vi "Nyquist Plot.vi"() -> ()   [LabVIEW 2018]
uses:
  <vilib>/addons/Control Design/_Model Construction/Model Typedefs.llb/CD Transfer Function Model (SISO).ctl
  <vilib>/addons/Control Design/_Model Construction/Data Typedefs.llb/CD frequency specs.ctl
  <vilib>/addons/Control Design/_Model Construction/Model Typedefs.llb/CD Transfer Function Model (MIMO).ctl
  <vilib>/addons/Control Design/_Model Construction/Model Typedefs.llb/CD General Elements.ctl
  <vilib>/addons/Control Design/_Utility/Rendering.llb/Rendering Transfer Function Options.ctl
  <vilib>/addons/Control Design/_Frequency Response Analysis/Frequency Response.llb/Frequency Response subVI/cd_Nyquist (Transfer Function).vi
  <vilib>/addons/Control Design/_Frequency Response Analysis/Frequency Response.llb/Frequency Response subVI/cd_Gain and Phase Margin (Transfer Function).vi
  <vilib>/addons/Control Design/_Utility/Model Viewer.llb/Model Viewer SubVI/cd_Draw Transfer Function Equation (TF).vi
  <vilib>/addons/Control Design/_Frequency Response Analysis/NI_CD_Frequency Response.lvlib
  <vilib>/addons/Control Design/_Model Construction/NI_LinSys_Data Typedefs.lvlib
  <vilib>/addons/Control Design/_Model Construction/NI_LinSys_Model Typedefs.lvlib
  <vilib>/addons/Control Design/_Utility/NI_CD_Model Viewer.lvlib
  <vilib>/addons/Control Design/_Utility/NI_LinSys_Rendering.lvlib
panel:
  out "nDelay":dbl
  out "P.M. Freq (rad/s)":dbl format="%#.2f"
  out "Phase Margin (rad)":dbl format="%#.2f"
  out "G.M. Freq (rad/s)":dbl format="%#.2f"
  out "Gain Margin":dbl format="%#.2f"
  out "Delay Margin":dbl format="%#.3f"
  out "D.M. Freq (rad/s)":dbl format="%#.2f"
  out "Forward Loop Transfer Function":picture
  in  "Transfer Function":T1[][](array[typedef]) {"delay" format="%.4f"; "Denominator" format="%#_6f"; "Numerator" format="%#.5f"}
  out "Nyquist Plot":cluster{"W":dbl[], "Magnitude":dbl[]}[](graph)
  # "Controls Board"
  # "Nyquist Plot"
  # "b0"
  # "b1"
  # "b2"
  # "b3"
  # "a0"
  # "a1"
  # "a2"
  # "a3"
  # "h"
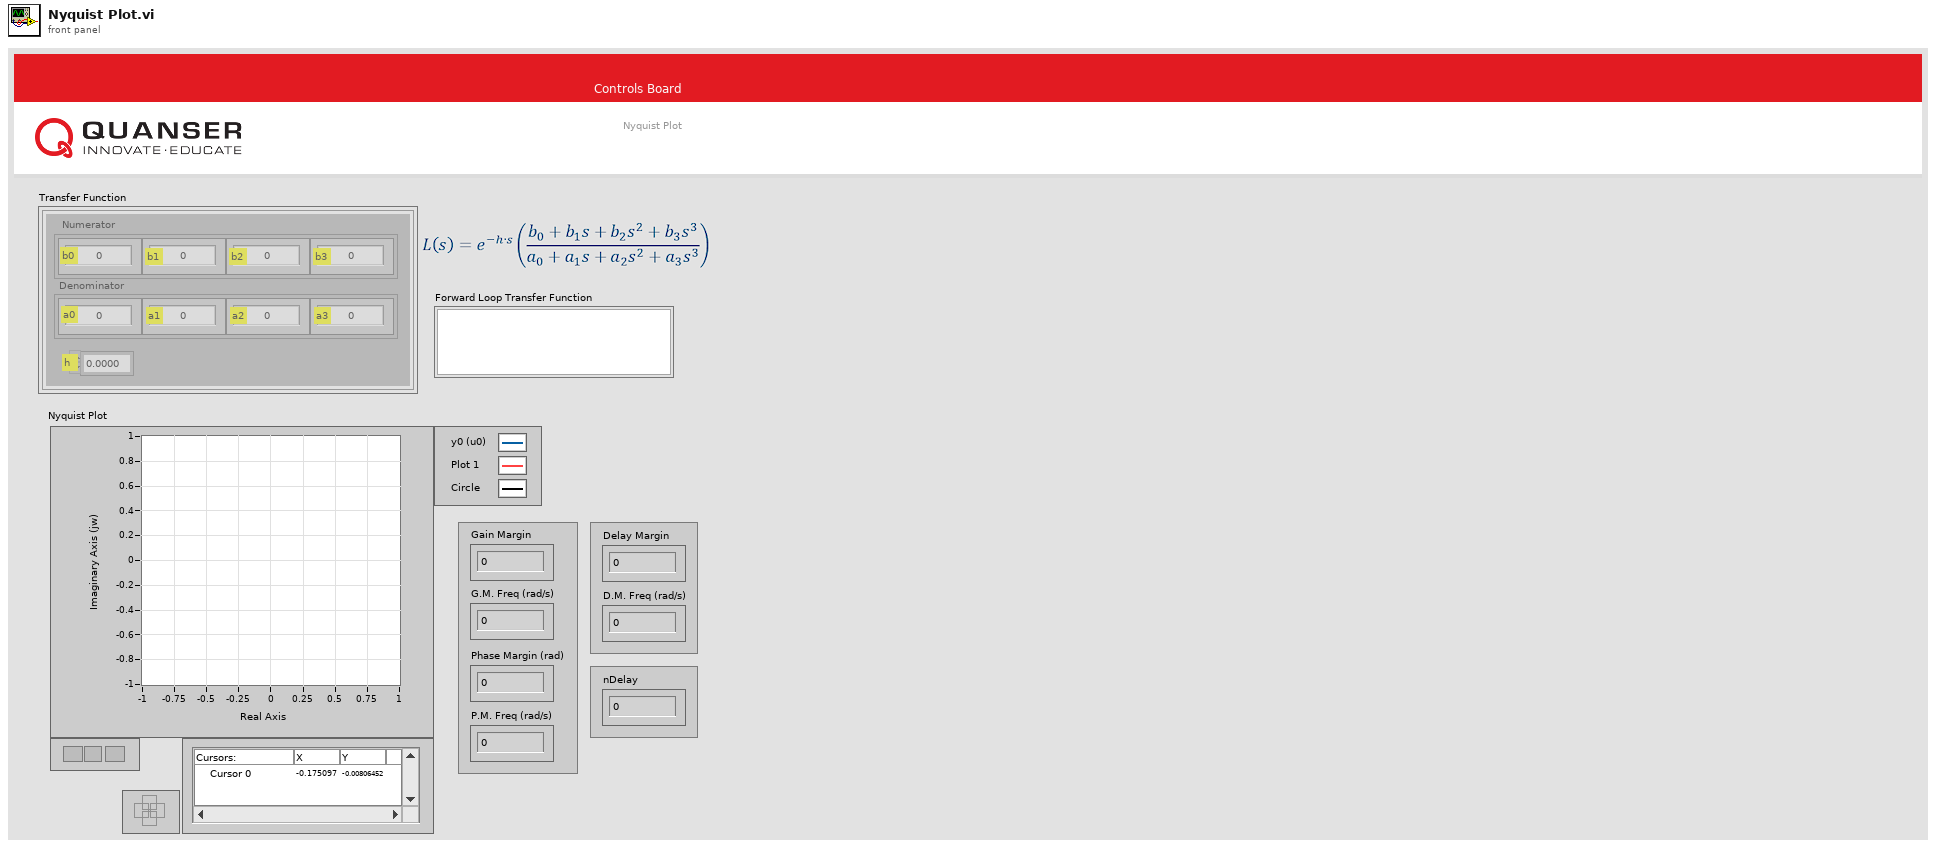
[diagram p1: front panel]
types:
  T1 = typedef "NI_LinSys_Model Typedefs.lvlib/CD Transfer Function Model (SISO).ctl" = cluster{"Numerator":dbl[], "Denominator":dbl[], "delay":dbl}
  T2 = typedef "NI_LinSys_Rendering.lvlib/Rendering Transfer Function Options.ctl" = u16
  T3 = typedef "NI_LinSys_Model Typedefs.lvlib/CD General Elements.ctl" = cluster{"Model name":string, "Input names":string[], "Output names":string[], "Input Delays":dbl[], "Output Delays":dbl[], "Sampling Time":dbl, "Notes":string}
  T4 = typedef "NI_LinSys_Model Typedefs.lvlib/CD Transfer Function Model (MIMO).ctl" = cluster{"properties":T3, "transfer function(s)":T1[][]}
  T5 = typedef "NI_LinSys_Data Typedefs.lvlib/CD frequency specs.ctl" = cluster{"Initial frequency":dbl, "Final frequency":dbl, "Minimum number of points":i32, "Frequency Unit":enum16{"Hz", "rad/s"}}
  T6 = typedef "NI_LinSys_Data Typedefs.lvlib/CD Margin Data.ctl" = cluster{"G.M. Frequency":dbl, "Gain Margin":dbl, "P.M. Frequency":dbl, "Phase Margin":dbl}
  T7 = typedef "NI_LinSys_Data Typedefs.lvlib/CD Delay Margin.ctl" = cluster{"D.M. Frequency":dbl, "Delay Margin":dbl}
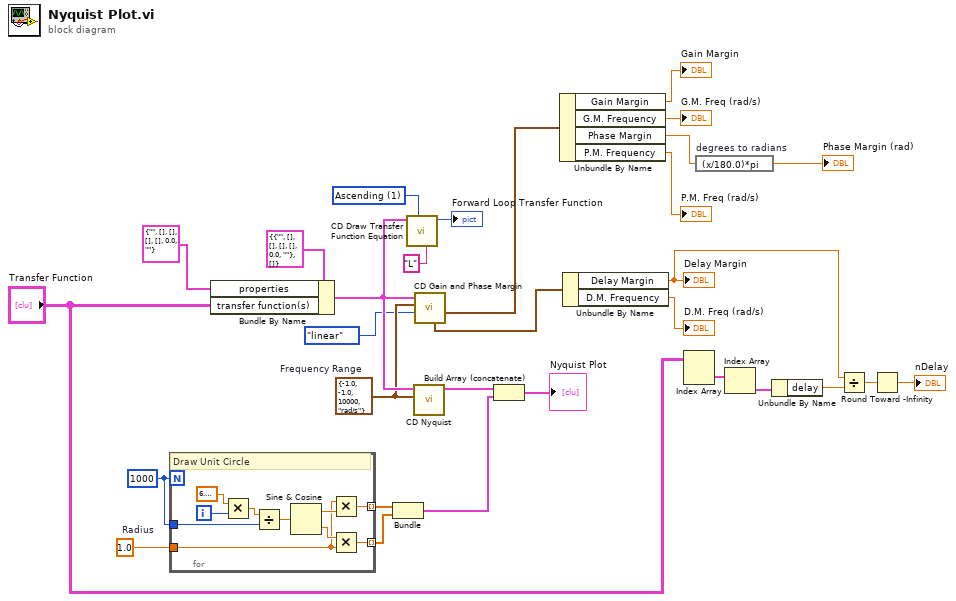
[diagram p0: block diagram]
diagram:
  w20 = T2 1 items=["Descending", "Ascending", "Negative Power"] ("Display Format")
  w24 = 1.0  # Radius
  w27 = 1000
  w18 = T5 {"Initial frequency"=-1.0, "Final frequency"=-1.0, "Minimum number of points"=10000, "Frequency Unit"=enum."rad/s"}  # Frequency Range
  n1 = for {
    N: w27 -> [_]
    tunnel: w27 -> [w38]
    tunnel: [w32] -> w26 mode=indexing
    tunnel: [w31] -> w25 mode=indexing
    tunnel: w24 -> [w33]
    i -> [w36]
    # "Draw Unit Circle"
    n2 = Multiply(x=6.283185307179586, y=w36) -> (x*y=w40:dbl)
    n3 = Divide(x=w40, y=w38) -> (x/y=w39:dbl)
    n4 = Sine & Cosine(0:w39) -> (1:w35:dbl, 2:w34:dbl)
    n5 = Multiply(x=w33, y=w35) -> (x*y=w32:dbl)
    n6 = Multiply(x=w34, y=w33) -> (x*y=w31:dbl)
  }
  n7 = Bundle By Name(cluster=T4 {"properties"={"Model name"="", "Input names"=[], "Output names"=[], "Input Delays"=[], "Output Delays"=[], "Sampling Time"=0.0, "Notes"=""}, "transfer function(s)"=[]} ("Transfer Function Model"), "properties"=T3 {"Model name"="", "Input names"=[], "Output names"=[], "Input Delays"=[], "Output Delays"=[], "Sampling Time"=0.0, "Notes"=""}, "transfer function(s)"="Transfer Function") -> (w19:T4)
  n8 = Bundle(w26, w25) -> (w22:cluster{dbl[], dbl[]})  [unwired: 1 in]
  n9 = call-poly <vilib>:"CD Draw Transfer Function Equation.vi"("Function Name (empty)"="L", "Display Format"=w20, "Transfer Function Model"=w19) -> ("Equation"=→"Forward Loop Transfer Function":picture)  [unwired: 6 in, 2 out]
  n10 = call-poly <vilib>:"CD Nyquist.vi"("Frequency Range"=w18, "Transfer Function Model"=w19) -> ("Nyquist Plot"=w23:cluster{"W":dbl[], "Magnitude":dbl[]}[])  [unwired: 7 in, 2 out]
  n11 = call-poly <vilib>:"CD Gain and Phase Margin.vi"("Magnitude Scale"=enum16{"linear", "dB"}."linear", "Frequency Range"=w18, "Transfer Function Model"=w19) -> ("Gain and Phase Margins"=w16:T6, "Delay Margin"=w15:T7)  [unwired: 4 in, 3 out]
  n12 = Build Array (concatenate)(w23, w22) -> (→"Nyquist Plot":cluster{"W":dbl[], "Magnitude":dbl[]}[])
  n13 = Unbundle By Name(w16) -> ("Gain Margin"=→"Gain Margin":dbl, "G.M. Frequency"=→"G.M. Freq (rad/s)":dbl, "Phase Margin"=w10:dbl, "P.M. Frequency"=→"P.M. Freq (rad/s)":dbl)
  n14 = Unbundle By Name(w15) -> ("Delay Margin"=w4:dbl, "D.M. Frequency"=→"D.M. Freq (rad/s)":dbl)
  "Delay Margin" <- w4
  n15 = Index Array(array="Transfer Function") -> (element=w7:T1[])  [unwired: 2 in]
  n16 = expression code="(x/180.0)*pi" "degrees to radians"(w10) -> (→"Phase Margin (rad)":dbl)
  n17 = Index Array(array=w7) -> (element=w6:T1)  [unwired: 1 in]
  n18 = Unbundle By Name(w6) -> ("delay"=w5:dbl)
  n19 = Divide(x=w4, y=w5) -> (x/y=w3:dbl)
  n20 = Round Toward -Infinity(1:w3) -> (0:→"nDelay":dbl)
